vi "Test Get Public API enum.vi"() -> ()   [LabVIEW 2019, in "Instrument.lvclass"]
uses:
  Instrument.lvclass
  Framework-Template/SMOs/Instrument.Framework-Template/Instrument.Framework-Template.lvclass
  C:/Users/patrick/Documents/GitHub/Instrument-Framework/lvsrc/Framework/Instrument/Instrument.lvclass
  b1b8d647-2e55-4445-909b-1706c674a77c.vi
  <vilib>/Utility/Data Type/Get Numeric Information.vi
panel:
  in  "s":bool
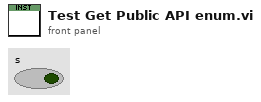
[diagram p1: front panel]
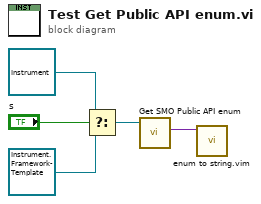
[diagram p0: block diagram]
diagram:
  n1 = Select(t=refnum<class "Instrument.lvclass"> refnum ("Instrument in"), s="s", f=refnum<class "Instrument.Framework-Template.lvclass"> refnum ("Instrument.Framework-Template.lvclass")) -> (s? t:f=w5:refnum<class "Instrument.lvclass">)
  n2 = call-dynamic "Get SMO Public API enum.vi"("Instrument in"=w5) -> ("Commands"=w1:variant)  [unwired: 8 in, 2 out]
  n3 = call "enum to string.vim"("enum in"=w1) -> ()  [unwired: 9 in, 2 out]
